vi "氨氮与上位机通讯.vi"   [LabVIEW 2016]
types:
  T1 = cluster{"因子编码":u32, "单位":u16, "标样参考值":sgl, "水样数据时间":timestamp, "水样实测值":sgl, "水样数据标识":string, "标样数据时间":timestamp, "标样实测值":sgl, "标样数据标识":string, "空白数据时间":timestamp, "空白实测值":sgl, "空白数据标识":string, "零点核查数据时间":timestamp, "零点核查实测值":sgl, "零点核查数据标识":string, "跨度核查数据时间":timestamp, "跨度核查实测值":sgl, "跨度核查数据标识":string, "加标回收数据时间":timestamp, "加标回收实测值":sgl, "加标回收数据标识":string, "平行样数据时间":timestamp, "平行样实测值":sgl, "平行样数据标识":string}
  T2 = cluster{"系统时间":timestamp, "工作状态":u16, "测量模式":u16, "告警代码":enum16{"无告警", "缺试剂告警", "缺水样告警", "缺蒸馏水告警", "缺标液告警", "仪表漏液告警", "标定异常告警", "超量程告警", "加热异常", "低试剂预警", "超上限告警", "超下限告警", "仪表内部其他异常", "滴定异常告警", "电极异常告警", "量程切换告警", "参数设置告警", "PH电极电位异常", "电导率电极异常", "浊度光度异常", "溶解氧电极异常", "溶解氧光强异常", "温度异常告警", "PH异常告警", "溶解氧异常告警", "电导率异常告警", "浊度异常告警", "叶绿素异常告警", "藻密度异常告警", "蓝绿藻异常告警", "ORP异常告警", "氨氮异常告警", "清洁刷异常告警", "SD卡异常告警", "蓝牙异常告警", "Wifi异常告警", "流程异常告警"}, "故障代码":enum16{"无故障", "电机故障", "温度故障", "通讯故障", "滴定故障"}, "日志代码":u16, "软件版本":u16, "F0":sgl, "F1":sgl, "F2":sgl, "F3":sgl, "T":sgl, "H":sgl, "id":u16, "flowid":u16, "量程":u16}
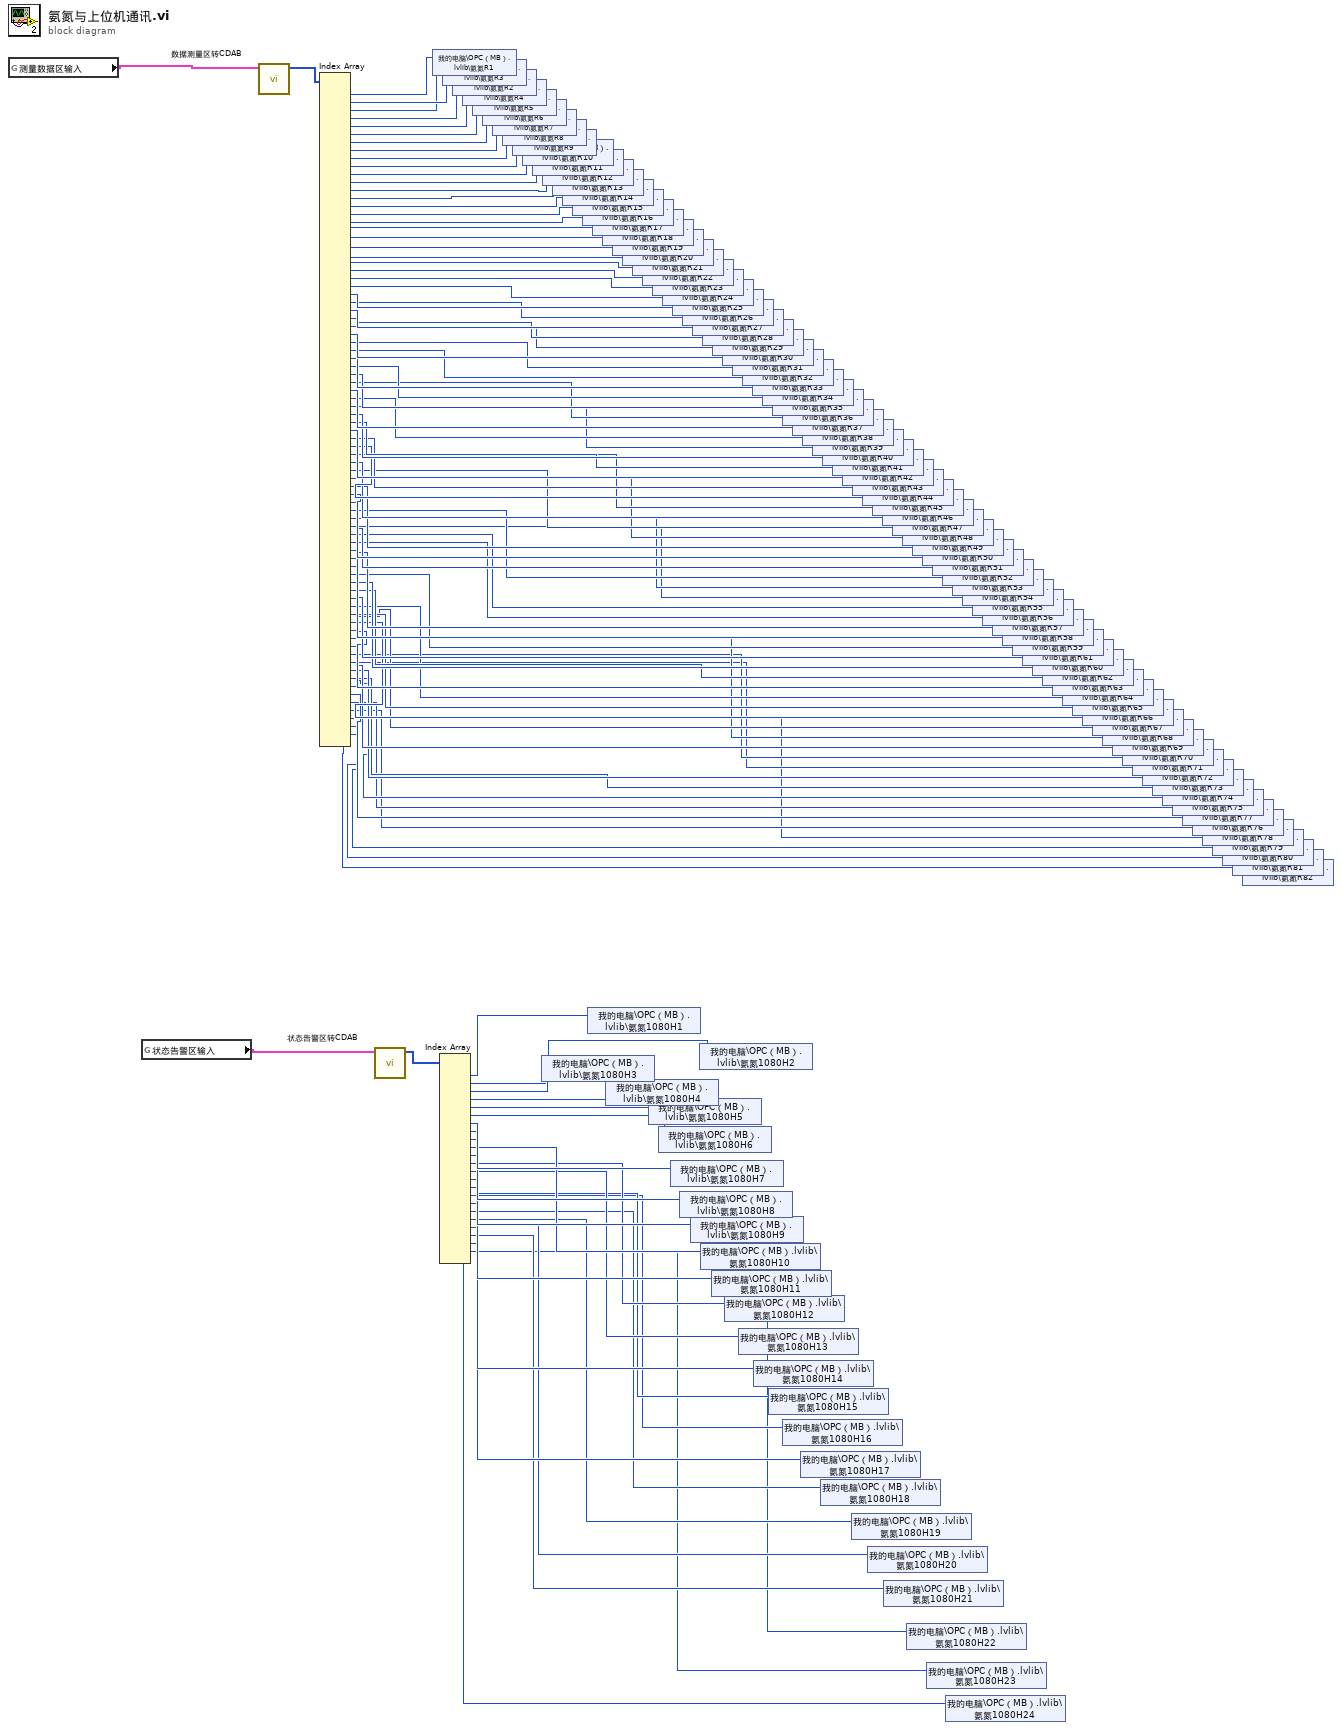
[diagram p0: block diagram]
diagram:
  n1 = global read "氨氮全局.vi" "测量数据区输入"() -> (w1:T1)
  n2 = global read "氨氮全局.vi" "状态告警区输入"() -> (w109:T2)
  n3 = call "数据测量区转CDAB.vi"("测量数据区"=w1) -> ("输出数组"=w84:u16[])  [unwired: 10 in]
  n4 = Index Array(array=w84) -> (element #1=w83:u16, element #2=w82:u16, element #3=w81:u16, element #4=w80:u16, element #5=w79:u16, element #6=w78:u16, element #7=w77:u16, element #8=w76:u16, element #9=w75:u16, element #10=w74:u16, element #11=w73:u16, element #12=w72:u16, element #13=w71:u16, element #14=w70:u16, element #15=w69:u16, element #16=w68:u16, element #17=w67:u16, element #18=w66:u16, element #19=w65:u16, element #20=w64:u16, element #21=w63:u16, element #22=w62:u16, element #23=w61:u16, element #24=w60:u16, element #25=w59:u16, element #26=w58:u16, element #27=w57:u16, element #28=w56:u16, element #29=w55:u16, element #30=w54:u16, element #31=w53:u16, element #32=w52:u16, element #33=w51:u16, element #34=w50:u16, element #35=w49:u16, element #36=w48:u16, element #37=w47:u16, element #38=w46:u16, element #39=w45:u16, element #40=w44:u16, element #41=w43:u16, element #42=w42:u16, element #43=w41:u16, element #44=w40:u16, element #45=w39:u16, element #46=w38:u16, element #47=w37:u16, element #48=w36:u16, element #49=w35:u16, element #50=w34:u16, element #51=w33:u16, element #52=w32:u16, element #53=w31:u16, element #54=w30:u16, element #55=w29:u16, element #56=w28:u16, element #57=w27:u16, element #58=w26:u16, element #59=w25:u16, element #60=w24:u16, element #61=w23:u16, element #62=w22:u16, element #63=w21:u16, element #64=w20:u16, element #65=w19:u16, element #66=w18:u16, element #67=w17:u16, element #68=w16:u16, element #69=w15:u16, element #70=w14:u16, element #71=w13:u16, element #72=w12:u16, element #73=w11:u16, element #74=w10:u16, element #75=w9:u16, element #76=w8:u16, element #77=w7:u16, element #78=w6:u16, element #79=w5:u16, element #80=w4:u16, element #81=w3:u16, element #82=w2:u16)  [unwired: 82 in]
  n5 = call "状态告警区转CDAB.vi"("状态告警区"=w109) -> ("输出数组"=w110:u16[])  [unwired: 10 in]
  n6 = shared-variable "我的电脑\\OPC（MB）.lvlib\\氨氮R1"(w83) -> ()  [unwired: 1 in, 1 out]
  n7 = Index Array(array=w110) -> (element #1=w108:u16, element #2=w85:u16, element #3=w107:u16, element #4=w106:u16, element #5=w105:u16, element #6=w104:u16, element #7=w103:u16, element #8=w102:u16, element #9=w101:u16, element #10=w100:u16, element #11=w99:u16, element #12=w98:u16, element #13=w97:u16, element #14=w96:u16, element #15=w95:u16, element #16=w94:u16, element #17=w93:u16, element #18=w92:u16, element #19=w91:u16, element #20=w90:u16, element #21=w89:u16, element #22=w88:u16, element #23=w87:u16, element #24=w86:u16)  [unwired: 24 in]
  n8 = shared-variable "我的电脑\\OPC（MB）.lvlib\\氨氮R3"(w81) -> ()  [unwired: 1 in, 1 out]
  n9 = shared-variable "我的电脑\\OPC（MB）.lvlib\\氨氮R2"(w82) -> ()  [unwired: 1 in, 1 out]
  n10 = shared-variable "我的电脑\\OPC（MB）.lvlib\\氨氮R4"(w80) -> ()  [unwired: 1 in, 1 out]
  n11 = shared-variable "我的电脑\\OPC（MB）.lvlib\\氨氮R5"(w79) -> ()  [unwired: 1 in, 1 out]
  n12 = shared-variable "我的电脑\\OPC（MB）.lvlib\\氨氮R6"(w78) -> ()  [unwired: 1 in, 1 out]
  n13 = shared-variable "我的电脑\\OPC（MB）.lvlib\\氨氮R7"(w77) -> ()  [unwired: 1 in, 1 out]
  n14 = shared-variable "我的电脑\\OPC（MB）.lvlib\\氨氮R8"(w76) -> ()  [unwired: 1 in, 1 out]
  n15 = shared-variable "我的电脑\\OPC（MB）.lvlib\\氨氮R9"(w75) -> ()  [unwired: 1 in, 1 out]
  n16 = shared-variable "我的电脑\\OPC（MB）.lvlib\\氨氮R10"(w74) -> ()  [unwired: 1 in, 1 out]
  n17 = shared-variable "我的电脑\\OPC（MB）.lvlib\\氨氮R11"(w73) -> ()  [unwired: 1 in, 1 out]
  n18 = shared-variable "我的电脑\\OPC（MB）.lvlib\\氨氮1080H3"(w107) -> ()  [unwired: 1 in, 1 out]
  n19 = shared-variable "我的电脑\\OPC（MB）.lvlib\\氨氮R12"(w72) -> ()  [unwired: 1 in, 1 out]
  n20 = shared-variable "我的电脑\\OPC（MB）.lvlib\\氨氮R13"(w71) -> ()  [unwired: 1 in, 1 out]
  n21 = shared-variable "我的电脑\\OPC（MB）.lvlib\\氨氮R14"(w70) -> ()  [unwired: 1 in, 1 out]
  n22 = shared-variable "我的电脑\\OPC（MB）.lvlib\\氨氮R15"(w69) -> ()  [unwired: 1 in, 1 out]
  n23 = shared-variable "我的电脑\\OPC（MB）.lvlib\\氨氮R16"(w68) -> ()  [unwired: 1 in, 1 out]
  n24 = shared-variable "我的电脑\\OPC（MB）.lvlib\\氨氮1080H1"(w108) -> ()  [unwired: 1 in, 1 out]
  n25 = shared-variable "我的电脑\\OPC（MB）.lvlib\\氨氮R17"(w67) -> ()  [unwired: 1 in, 1 out]
  n26 = shared-variable "我的电脑\\OPC（MB）.lvlib\\氨氮R18"(w66) -> ()  [unwired: 1 in, 1 out]
  n27 = shared-variable "我的电脑\\OPC（MB）.lvlib\\氨氮1080H4"(w106) -> ()  [unwired: 1 in, 1 out]
  n28 = shared-variable "我的电脑\\OPC（MB）.lvlib\\氨氮R19"(w65) -> ()  [unwired: 1 in, 1 out]
  n29 = shared-variable "我的电脑\\OPC（MB）.lvlib\\氨氮R20"(w64) -> ()  [unwired: 1 in, 1 out]
  n30 = shared-variable "我的电脑\\OPC（MB）.lvlib\\氨氮R21"(w63) -> ()  [unwired: 1 in, 1 out]
  n31 = shared-variable "我的电脑\\OPC（MB）.lvlib\\氨氮R22"(w62) -> ()  [unwired: 1 in, 1 out]
  n32 = shared-variable "我的电脑\\OPC（MB）.lvlib\\氨氮1080H5"(w105) -> ()  [unwired: 1 in, 1 out]
  n33 = shared-variable "我的电脑\\OPC（MB）.lvlib\\氨氮R23"(w61) -> ()  [unwired: 1 in, 1 out]
  n34 = shared-variable "我的电脑\\OPC（MB）.lvlib\\氨氮1080H6"(w104) -> ()  [unwired: 1 in, 1 out]
  n35 = shared-variable "我的电脑\\OPC（MB）.lvlib\\氨氮R24"(w60) -> ()  [unwired: 1 in, 1 out]
  n36 = shared-variable "我的电脑\\OPC（MB）.lvlib\\氨氮1080H7"(w103) -> ()  [unwired: 1 in, 1 out]
  n37 = shared-variable "我的电脑\\OPC（MB）.lvlib\\氨氮R25"(w59) -> ()  [unwired: 1 in, 1 out]
  n38 = shared-variable "我的电脑\\OPC（MB）.lvlib\\氨氮1080H8"(w102) -> ()  [unwired: 1 in, 1 out]
  n39 = shared-variable "我的电脑\\OPC（MB）.lvlib\\氨氮R26"(w58) -> ()  [unwired: 1 in, 1 out]
  n40 = shared-variable "我的电脑\\OPC（MB）.lvlib\\氨氮1080H9"(w101) -> ()  [unwired: 1 in, 1 out]
  n41 = shared-variable "我的电脑\\OPC（MB）.lvlib\\氨氮R27"(w57) -> ()  [unwired: 1 in, 1 out]
  n42 = shared-variable "我的电脑\\OPC（MB）.lvlib\\氨氮1080H2"(w85) -> ()  [unwired: 1 in, 1 out]
  n43 = shared-variable "我的电脑\\OPC（MB）.lvlib\\氨氮1080H10"(w100) -> ()  [unwired: 1 in, 1 out]
  n44 = shared-variable "我的电脑\\OPC（MB）.lvlib\\氨氮R28"(w56) -> ()  [unwired: 1 in, 1 out]
  n45 = shared-variable "我的电脑\\OPC（MB）.lvlib\\氨氮1080H11"(w99) -> ()  [unwired: 1 in, 1 out]
  n46 = shared-variable "我的电脑\\OPC（MB）.lvlib\\氨氮R29"(w55) -> ()  [unwired: 1 in, 1 out]
  n47 = shared-variable "我的电脑\\OPC（MB）.lvlib\\氨氮R30"(w54) -> ()  [unwired: 1 in, 1 out]
  n48 = shared-variable "我的电脑\\OPC（MB）.lvlib\\氨氮1080H12"(w98) -> ()  [unwired: 1 in, 1 out]
  n49 = shared-variable "我的电脑\\OPC（MB）.lvlib\\氨氮R31"(w53) -> ()  [unwired: 1 in, 1 out]
  n50 = shared-variable "我的电脑\\OPC（MB）.lvlib\\氨氮1080H13"(w97) -> ()  [unwired: 1 in, 1 out]
  n51 = shared-variable "我的电脑\\OPC（MB）.lvlib\\氨氮R32"(w52) -> ()  [unwired: 1 in, 1 out]
  n52 = shared-variable "我的电脑\\OPC（MB）.lvlib\\氨氮R33"(w51) -> ()  [unwired: 1 in, 1 out]
  n53 = shared-variable "我的电脑\\OPC（MB）.lvlib\\氨氮1080H14"(w96) -> ()  [unwired: 1 in, 1 out]
  n54 = shared-variable "我的电脑\\OPC（MB）.lvlib\\氨氮R34"(w50) -> ()  [unwired: 1 in, 1 out]
  n55 = shared-variable "我的电脑\\OPC（MB）.lvlib\\氨氮1080H15"(w95) -> ()  [unwired: 1 in, 1 out]
  n56 = shared-variable "我的电脑\\OPC（MB）.lvlib\\氨氮R35"(w49) -> ()  [unwired: 1 in, 1 out]
  n57 = shared-variable "我的电脑\\OPC（MB）.lvlib\\氨氮R36"(w48) -> ()  [unwired: 1 in, 1 out]
  n58 = shared-variable "我的电脑\\OPC（MB）.lvlib\\氨氮1080H16"(w94) -> ()  [unwired: 1 in, 1 out]
  n59 = shared-variable "我的电脑\\OPC（MB）.lvlib\\氨氮R37"(w47) -> ()  [unwired: 1 in, 1 out]
  n60 = shared-variable "我的电脑\\OPC（MB）.lvlib\\氨氮1080H17"(w93) -> ()  [unwired: 1 in, 1 out]
  n61 = shared-variable "我的电脑\\OPC（MB）.lvlib\\氨氮R38"(w46) -> ()  [unwired: 1 in, 1 out]
  n62 = shared-variable "我的电脑\\OPC（MB）.lvlib\\氨氮R39"(w45) -> ()  [unwired: 1 in, 1 out]
  n63 = shared-variable "我的电脑\\OPC（MB）.lvlib\\氨氮1080H18"(w92) -> ()  [unwired: 1 in, 1 out]
  n64 = shared-variable "我的电脑\\OPC（MB）.lvlib\\氨氮R40"(w44) -> ()  [unwired: 1 in, 1 out]
  n65 = shared-variable "我的电脑\\OPC（MB）.lvlib\\氨氮R41"(w43) -> ()  [unwired: 1 in, 1 out]
  n66 = shared-variable "我的电脑\\OPC（MB）.lvlib\\氨氮R42"(w42) -> ()  [unwired: 1 in, 1 out]
  n67 = shared-variable "我的电脑\\OPC（MB）.lvlib\\氨氮1080H19"(w91) -> ()  [unwired: 1 in, 1 out]
  n68 = shared-variable "我的电脑\\OPC（MB）.lvlib\\氨氮R43"(w41) -> ()  [unwired: 1 in, 1 out]
  n69 = shared-variable "我的电脑\\OPC（MB）.lvlib\\氨氮R44"(w40) -> ()  [unwired: 1 in, 1 out]
  n70 = shared-variable "我的电脑\\OPC（MB）.lvlib\\氨氮1080H20"(w90) -> ()  [unwired: 1 in, 1 out]
  n71 = shared-variable "我的电脑\\OPC（MB）.lvlib\\氨氮R45"(w39) -> ()  [unwired: 1 in, 1 out]
  n72 = shared-variable "我的电脑\\OPC（MB）.lvlib\\氨氮R46"(w38) -> ()  [unwired: 1 in, 1 out]
  n73 = shared-variable "我的电脑\\OPC（MB）.lvlib\\氨氮1080H21"(w89) -> ()  [unwired: 1 in, 1 out]
  n74 = shared-variable "我的电脑\\OPC（MB）.lvlib\\氨氮R47"(w37) -> ()  [unwired: 1 in, 1 out]
  n75 = shared-variable "我的电脑\\OPC（MB）.lvlib\\氨氮R48"(w36) -> ()  [unwired: 1 in, 1 out]
  n76 = shared-variable "我的电脑\\OPC（MB）.lvlib\\氨氮1080H22"(w88) -> ()  [unwired: 1 in, 1 out]
  n77 = shared-variable "我的电脑\\OPC（MB）.lvlib\\氨氮R49"(w35) -> ()  [unwired: 1 in, 1 out]
  n78 = shared-variable "我的电脑\\OPC（MB）.lvlib\\氨氮R50"(w34) -> ()  [unwired: 1 in, 1 out]
  n79 = shared-variable "我的电脑\\OPC（MB）.lvlib\\氨氮1080H23"(w87) -> ()  [unwired: 1 in, 1 out]
  n80 = shared-variable "我的电脑\\OPC（MB）.lvlib\\氨氮R51"(w33) -> ()  [unwired: 1 in, 1 out]
  n81 = shared-variable "我的电脑\\OPC（MB）.lvlib\\氨氮R52"(w32) -> ()  [unwired: 1 in, 1 out]
  n82 = shared-variable "我的电脑\\OPC（MB）.lvlib\\氨氮1080H24"(w86) -> ()  [unwired: 1 in, 1 out]
  n83 = shared-variable "我的电脑\\OPC（MB）.lvlib\\氨氮R53"(w31) -> ()  [unwired: 1 in, 1 out]
  n84 = shared-variable "我的电脑\\OPC（MB）.lvlib\\氨氮R54"(w30) -> ()  [unwired: 1 in, 1 out]
  n85 = shared-variable "我的电脑\\OPC（MB）.lvlib\\氨氮R55"(w29) -> ()  [unwired: 1 in, 1 out]
  n86 = shared-variable "我的电脑\\OPC（MB）.lvlib\\氨氮R56"(w28) -> ()  [unwired: 1 in, 1 out]
  n87 = shared-variable "我的电脑\\OPC（MB）.lvlib\\氨氮R57"(w27) -> ()  [unwired: 1 in, 1 out]
  n88 = shared-variable "我的电脑\\OPC（MB）.lvlib\\氨氮R58"(w26) -> ()  [unwired: 1 in, 1 out]
  n89 = shared-variable "我的电脑\\OPC（MB）.lvlib\\氨氮R59"(w25) -> ()  [unwired: 1 in, 1 out]
  n90 = shared-variable "我的电脑\\OPC（MB）.lvlib\\氨氮R61"(w23) -> ()  [unwired: 1 in, 1 out]
  n91 = shared-variable "我的电脑\\OPC（MB）.lvlib\\氨氮R60"(w24) -> ()  [unwired: 1 in, 1 out]
  n92 = shared-variable "我的电脑\\OPC（MB）.lvlib\\氨氮R62"(w22) -> ()  [unwired: 1 in, 1 out]
  n93 = shared-variable "我的电脑\\OPC（MB）.lvlib\\氨氮R63"(w21) -> ()  [unwired: 1 in, 1 out]
  n94 = shared-variable "我的电脑\\OPC（MB）.lvlib\\氨氮R64"(w20) -> ()  [unwired: 1 in, 1 out]
  n95 = shared-variable "我的电脑\\OPC（MB）.lvlib\\氨氮R65"(w19) -> ()  [unwired: 1 in, 1 out]
  n96 = shared-variable "我的电脑\\OPC（MB）.lvlib\\氨氮R66"(w18) -> ()  [unwired: 1 in, 1 out]
  n97 = shared-variable "我的电脑\\OPC（MB）.lvlib\\氨氮R67"(w17) -> ()  [unwired: 1 in, 1 out]
  n98 = shared-variable "我的电脑\\OPC（MB）.lvlib\\氨氮R68"(w16) -> ()  [unwired: 1 in, 1 out]
  n99 = shared-variable "我的电脑\\OPC（MB）.lvlib\\氨氮R69"(w15) -> ()  [unwired: 1 in, 1 out]
  n100 = shared-variable "我的电脑\\OPC（MB）.lvlib\\氨氮R70"(w14) -> ()  [unwired: 1 in, 1 out]
  n101 = shared-variable "我的电脑\\OPC（MB）.lvlib\\氨氮R71"(w13) -> ()  [unwired: 1 in, 1 out]
  n102 = shared-variable "我的电脑\\OPC（MB）.lvlib\\氨氮R72"(w12) -> ()  [unwired: 1 in, 1 out]
  n103 = shared-variable "我的电脑\\OPC（MB）.lvlib\\氨氮R73"(w11) -> ()  [unwired: 1 in, 1 out]
  n104 = shared-variable "我的电脑\\OPC（MB）.lvlib\\氨氮R74"(w10) -> ()  [unwired: 1 in, 1 out]
  n105 = shared-variable "我的电脑\\OPC（MB）.lvlib\\氨氮R75"(w9) -> ()  [unwired: 1 in, 1 out]
  n106 = shared-variable "我的电脑\\OPC（MB）.lvlib\\氨氮R77"(w7) -> ()  [unwired: 1 in, 1 out]
  n107 = shared-variable "我的电脑\\OPC（MB）.lvlib\\氨氮R76"(w8) -> ()  [unwired: 1 in, 1 out]
  n108 = shared-variable "我的电脑\\OPC（MB）.lvlib\\氨氮R78"(w6) -> ()  [unwired: 1 in, 1 out]
  n109 = shared-variable "我的电脑\\OPC（MB）.lvlib\\氨氮R79"(w5) -> ()  [unwired: 1 in, 1 out]
  n110 = shared-variable "我的电脑\\OPC（MB）.lvlib\\氨氮R80"(w4) -> ()  [unwired: 1 in, 1 out]
  n111 = shared-variable "我的电脑\\OPC（MB）.lvlib\\氨氮R81"(w3) -> ()  [unwired: 1 in, 1 out]
  n112 = shared-variable "我的电脑\\OPC（MB）.lvlib\\氨氮R82"(w2) -> ()  [unwired: 1 in, 1 out]
